vi "01pixmap.vi"(1 "Input pixmap":u8[][](array[numeric])) -> (0 "0/1 pixmap":i32[][](array[numeric]))   [LabVIEW 2016]
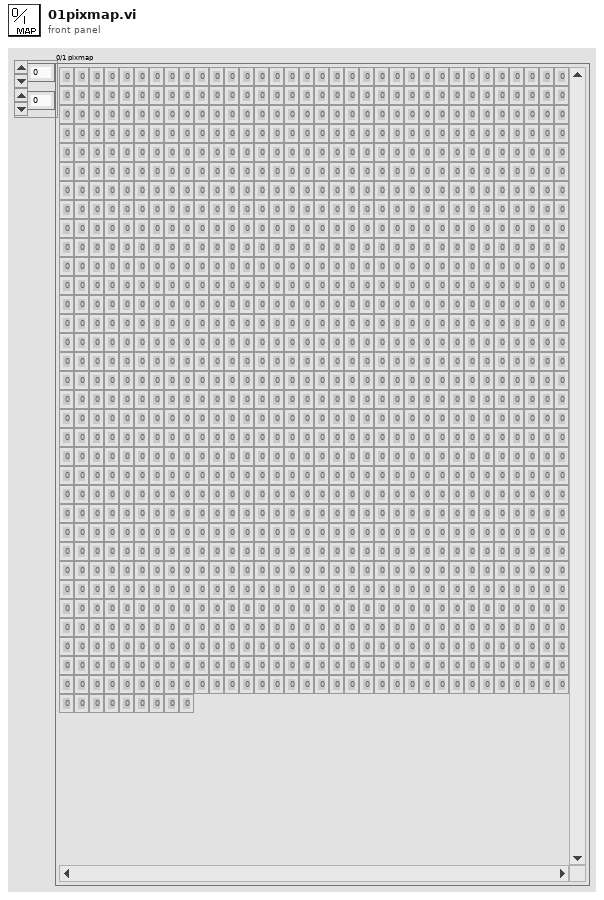
[diagram p1: front panel]
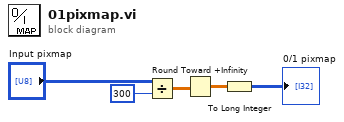
[diagram p0: block diagram]
diagram:
  n1 = Divide(x="Input pixmap", y=300) -> (x/y=w3:dbl[][])
  n2 = Round Toward +Infinity(x=w3) -> (ceil(x): smallest int >= x=w4:dbl[][])
  n3 = To Long Integer(number=w4) -> (32bit integer=→"0/1 pixmap":i32[][])
